vi "TD_Open_Connection.vi"() -> ()   [LabVIEW 2018]
uses:
  <vilib>/httpClient/ClientHandle.ctl
  <vilib>/httpClient/LabVIEWHTTPClient.lvlib
panel:
  out "HTTP TekDrive Session":T1
  out "Error Out":errorcluster
  in  "Error In":errorcluster
  in  "Access Key":string
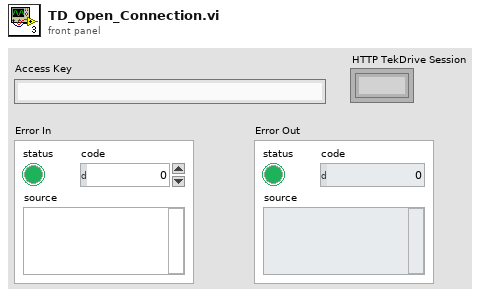
[diagram p1: front panel]
types:
  T1 = typedef "LabVIEWHTTPClient.lvlib/ClientHandle.ctl" = refnum<k1>
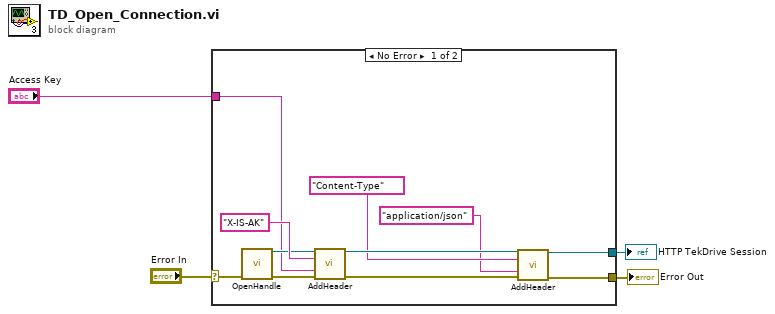
[diagram p0: block diagram]
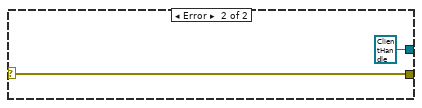
[diagram p2: hidden frame]
diagram:
  n1 = case shown="No Error" "Error In" {
    selector: "Error In" -> [w15 w17]
    tunnel: "Access Key" -> [w11 _]
    tunnel: [w6 T1 refnum ("client handle out")] -> w1
    tunnel: [w5 w17] -> w2
    frame No Error {
      n2 = call <vilib>:"OpenHandle.vi"("error in (no error)"=w15) -> ("client handle out"=w12:T1, "error out"=w14:errorcluster)  [unwired: 13 in]
      n3 = call <vilib>:"AddHeader.vi"("client handle"=w12, "header"="X-IS-AK" ("Access Key"), "value"=w11, "error in (no error)"=w14) -> ("client handle out"=w10:T1, "error out"=w9:errorcluster)  [unwired: 10 in]
      n4 = call <vilib>:"AddHeader.vi"("client handle"=w10, "header"="Content-Type", "value"="application/json", "error in (no error)"=w9) -> ("client handle out"=w6:T1, "error out"=w5:errorcluster)  [unwired: 10 in]
    }
    frame Error {
    }
  }
  "Error Out" <- w2
  "HTTP TekDrive Session" <- w1
